vi "Find GUID Down.vi"(8 "error in (no error)":errorcluster, 9 "Find Alll?":bool, 10 "BaseNdType":refnum<k24>, 11 "GUID":string) -> (0 "error out":errorcluster, 1 "FindNodeMatchGUID":refnum<k24>[](array[refnum]), 2 "BaseNdType":refnum<k24>, 4 "Found":bool)   [LabVIEW 2014]
uses:
  NationalInstruments.VeriStand.SystemStorage
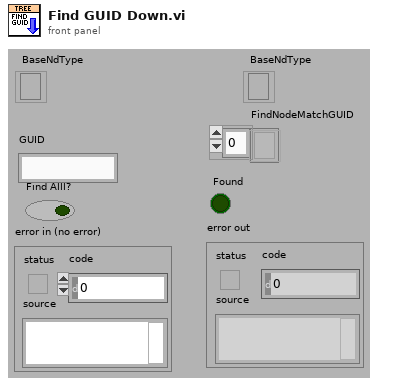
[diagram p1: front panel]
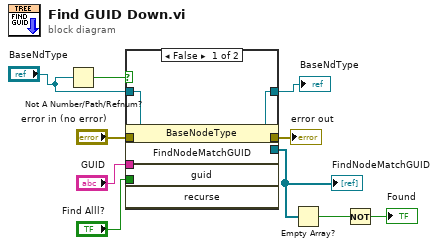
[diagram p0: block diagram]
diagram:
  n1 = Not A Number/Path/Refnum?(number/path/refnum="BaseNdType") -> (NaN/Path/Refnum?=w3:bool)
  n2 = case shown="False" w3 {
    tunnel: [w17 _] -> w8
    tunnel: "Find Alll?" -> [w16 _]
    tunnel: "GUID" -> [w15 _]
    tunnel: [w14 w19] -> w5
    tunnel: [w13 w18] -> w1
    tunnel: "error in (no error)" -> [w12 w19]
    tunnel: "BaseNdType" -> [w11 w18]
    frame False {
      n3 = invoke class="BaseNodeType" method="FindNodeMatchGUID"(reference=w11, error in=w12, "guid"=w15, "recurse"=w16) -> (reference out=w13:refnum<k24>, error out=w14:errorcluster, "FindNodeMatchGUID"=w17:refnum<k24>[])  [unwired: 1 in, 2 out]
    }
    frame True {
    }
  }
  "error out" <- w5
  "FindNodeMatchGUID" <- w8
  "BaseNdType" <- w1
  n4 = Empty Array?(array=w8) -> (empty?=w9:bool)
  n5 = Not(x=w9) -> (.not. x?=→"Found":bool)
